vi "DSF.Engine.Transceiver.Response.Receive.vi"(8 "error in (no error)":errorcluster, 9 "timeout in ms (0)":i32 format="%d ms", 11 "Transceiver Thread in":refnum<class "DSF.Engine.Interface.Transceiver.lvclass">) -> (0 "error out":errorcluster, 1 "timed out?":bool, 2 "response":T1, 3 "Transceiver Thread out":refnum<class "DSF.Engine.Interface.Transceiver.lvclass">)   [LabVIEW 2017, in "DSF.Engine.lvlib" / "DSF.Engine.Transceiver Thread.lvclass"]
uses:
  DSF.Engine.Transceiver Thread.lvclass
  Interface/DSF.Engine.Interface.Transceiver.lvclass
  Interface/DSF.Engine.Interface.Transceiver.Response Data.ctl
  Interface/DSF.Engine.Interface.Transceiver.Response.ctl
  Interface/DSF.Engine.Interface.Transceiver.Response Parameters.ctl
  Interface/DSF.Engine.Interface.Transceiver.Read.Response.vi
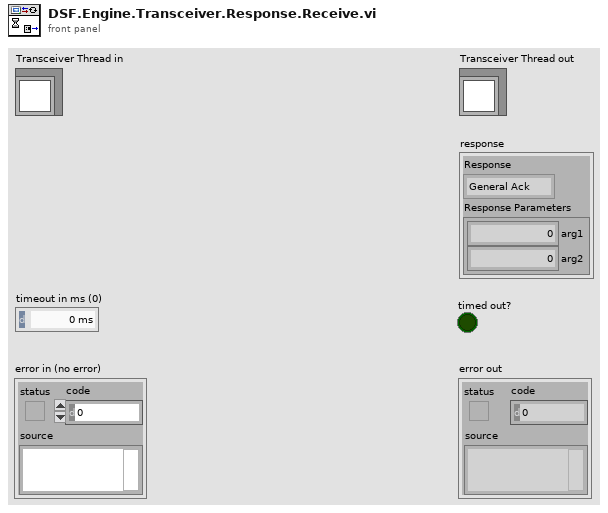
[diagram p1: front panel]
types:
  T1 = typedef "DSF.Engine.lvlib/DSF.Engine.Interface.Transceiver.lvclass/DSF.Engine.Interface.Transceiver.Response Data.ctl" = cluster{"Response":T2, "Response Parameters":T3}
  T2 = typedef "DSF.Engine.lvlib/DSF.Engine.Interface.Transceiver.lvclass/DSF.Engine.Interface.Transceiver.Response.ctl" = enum8{"General Ack", "Shutting Down"}
  T3 = typedef "DSF.Engine.lvlib/DSF.Engine.Interface.Transceiver.lvclass/DSF.Engine.Interface.Transceiver.Response Parameters.ctl" = cluster{"arg1":u64, "arg2":u64}
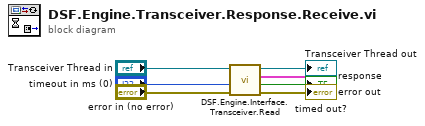
[diagram p0: block diagram]
diagram:
  n1 = call-poly "DSF.Engine.Interface.Transceiver.Read.vi"("error in (no error)"="error in (no error)", "timeout in ms (0)"="timeout in ms (0)", "Transceiver Interface in"="Transceiver Thread in") -> ("error out"=→"error out":errorcluster, "empty?"=→"timed out?":bool, "response"=→"response":T1, "Transceiver Interface out"=→"Transceiver Thread out":refnum<class "DSF.Engine.Interface.Transceiver.lvclass">)  [unwired: 4 in, 1 out]
